vi "attributes-test.vi"(8 "error in (no error)":errorcluster) -> (0 "error out":errorcluster)   [LabVIEW 2013]
uses:
  src/Support/Attribute.Identity/Attribute.Identity.lvclass/Attribute.Identity.ctl
  <vilib>/addons/_JKI Toolkits/Caraya/classes/Test/Test.lvclass
  <vilib>/addons/_JKI Toolkits/Caraya/classes/Assert/Assert.lvclass
  src/Support/Attribute.Identity/Attribute.Identity.lvclass
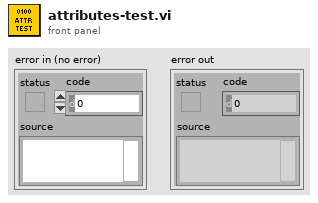
[diagram p1: front panel]
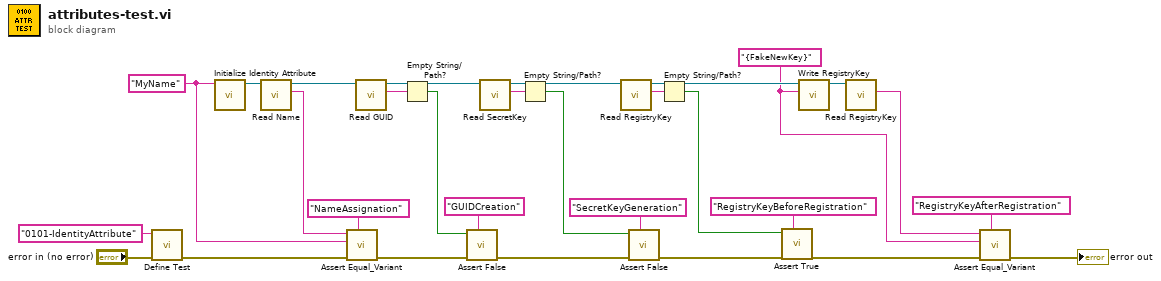
[diagram p0: block diagram]
diagram:
  w3 = "{FakeNewKey}" ("Label (VI Title)")
  w20 = "MyName" ("Name")
  n1 = call <vilib>:"Define Test.vi"("error in (no error)"="error in (no error)", "Label (VI Title)"="0101-IdentityAttribute") -> ("error out"=w28:errorcluster)  [unwired: 9 in]
  n2 = call "Initialize Identity Attribute.vi"("Name"=w20) -> ("Attribute.Identity"=w25:refnum<class "Attribute.Identity.lvclass">)  [unwired: 10 in]
  n3 = call "Read Name.vi"("Attribute.Identity in"=w25) -> ("Name"=w21:string, "Attribute.Identity out"=w24:refnum<class "Attribute.Identity.lvclass">)  [unwired: 8 in, 1 out]
  n4 = call <vilib>:"Assert Equal_Variant.vi"("Label"="NameAssignation" ("Label (VI Title)"), "error in (no error)"=w28, "Y"=w20, "X"=w21) -> ("error out"=w18:errorcluster)  [unwired: 7 in]
  n5 = call "Read GUID.vi"("Attribute.Identity in"=w24) -> ("GUID"=w19:string, "Attribute.Identity out"=w23:refnum<class "Attribute.Identity.lvclass">)  [unwired: 8 in, 1 out]
  n6 = Empty String/Path?(string/path=w19) -> (empty?=w17:bool)
  n7 = call <vilib>:"Assert False.vi"("Label"="GUIDCreation" ("Label (VI Title)"), "error in (no error)"=w18, "False?"=w17) -> ("error out"=w15:errorcluster)  [unwired: 8 in]
  n8 = call "Read SecretKey.vi"("Attribute.Identity in"=w23) -> ("SecretKey"=w13:string, "Attribute.Identity out"=w11:refnum<class "Attribute.Identity.lvclass">)  [unwired: 8 in, 1 out]
  n9 = Empty String/Path?(string/path=w13) -> (empty?=w12:bool)
  n10 = call "Read RegistryKey.vi"("Attribute.Identity in"=w11) -> ("RegistryKey"=w9:string, "Attribute.Identity out"=w10:refnum<class "Attribute.Identity.lvclass">)  [unwired: 8 in, 1 out]
  n11 = call <vilib>:"Assert False.vi"("Label"="SecretKeyGeneration" ("Label (VI Title)"), "error in (no error)"=w15, "False?"=w12) -> ("error out"=w7:errorcluster)  [unwired: 8 in]
  n12 = Empty String/Path?(string/path=w9) -> (empty?=w6:bool)
  n13 = call <vilib>:"Assert True.vi"("Label"="RegistryKeyBeforeRegistration" ("Label (VI Title)"), "error in (no error)"=w7, "True?"=w6) -> ("error out"=w5:errorcluster)  [unwired: 8 in]
  n14 = call "Write RegistryKey.vi"("RegistryKey"=w3, "Attribute.Identity in"=w10) -> ("Attribute.Identity out"=w22:refnum<class "Attribute.Identity.lvclass">)  [unwired: 8 in, 1 out]
  n15 = call "Read RegistryKey.vi"("Attribute.Identity in"=w22) -> ("RegistryKey"=w4:string)  [unwired: 8 in, 2 out]
  n16 = call <vilib>:"Assert Equal_Variant.vi"("Label"="RegistryKeyAfterRegistration" ("Label (VI Title)"), "error in (no error)"=w5, "Y"=w3, "X"=w4) -> ("error out"=→"error out":errorcluster)  [unwired: 7 in]
